vi "SParmSetup_v1.1.vi"(0 "VISA IN":refnum<visa-resource-name>="GPIB0::16::INSTR", 1 "Start Frequency":dbl=10000000.0, 2 "Stop Frequency":dbl=26400000000.0, 3 "Filename":string="MY_MEAS", 5 "Average?":bool=TRUE, 6 "AVG Factor":i32=5, 7 "error in":errorcluster, 8 "Autoscale?":bool, 9 "Trace":i32=1, 10 "Points":dbl=201.0, 11 "Window":i32=1, 12 "IF BW":dbl=1000.0, 13 "Channel":i32=1, 14 "Format":string(combo)="MLINear", 15 "Sweep Type":string(combo)="LINear", 17 "Power Level":dbl=-10.0, 19 "CW Frq.":dbl=1000000000.0, 26 "CW Points":dbl=1.0) -> (20 "VISA Out":refnum<visa-resource-name>="GPIB0::16::INSTR", 27 "error out":errorcluster)   [LabVIEW 2018]
panel:
  in  "Ref Position":i32
  in  "Ref Level":i32
  in  "Scale Per Division":i32=10
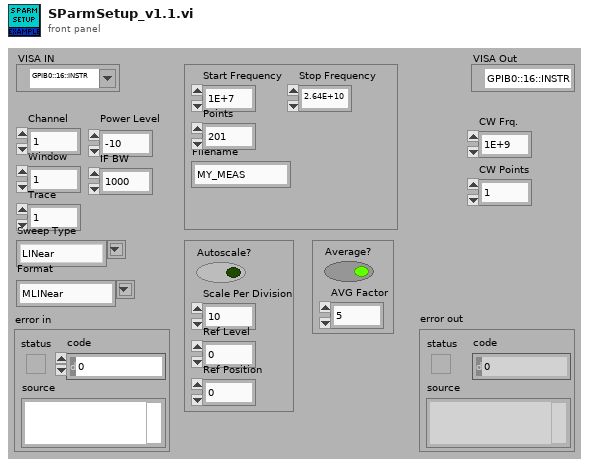
[diagram p1: front panel]
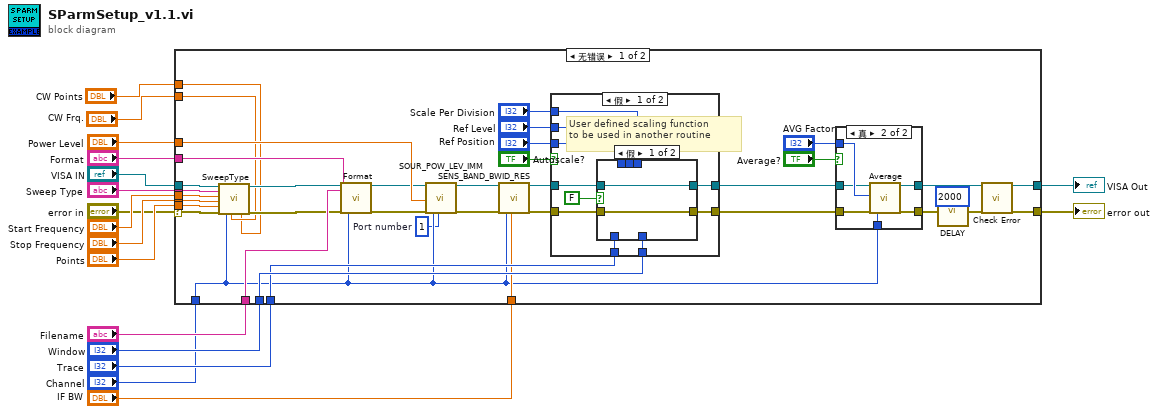
[diagram p0: block diagram]
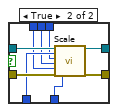
[diagram p3: hidden frame]
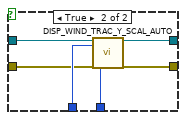
[diagram p4: hidden frame]
diagram:
  n1 = case shown="无错误" "error in" {
    selector: "error in" -> [w23 w92]
    tunnel: [w55 w91] -> w17
    tunnel: [w54 w92] -> w16
    tunnel: "Stop Frequency" -> [w53 _]
    tunnel: "Points" -> [w52 _]
    tunnel: "Sweep Type" -> [w51 _]
    tunnel: "Start Frequency" -> [w50 _]
    tunnel: "Window" -> [w49 _]
    tunnel: "Trace" -> [w48 _]
    tunnel: "VISA IN" -> [w36 w91]
    tunnel: "Power Level" -> [w34 _]
    tunnel: "IF BW" -> [w29 _]
    tunnel: "Filename" -> [w26 _]
    tunnel: "Channel" -> [w25 _]
    tunnel: "Format" -> [w24 _]
    tunnel: "CW Frq." -> [w19 _]
    tunnel: "CW Points" -> [w18 _]
    frame No Error {
      w22 = 1  # Port number
      n2 = call "SweepType.vi"("VISA IN"=w36, "Sweep Type"=w51, "Start Frq."=w50, "Stop Frq."=w53, 4:"Points"=w52, "error in"=w23, "Channel"=w25, "CW Frq."=w19, 13:"Points"=w18) -> ("VISA Out"=w21:refnum<visa-resource-name>, "error out"=w20:errorcluster)  [unwired: 9 in]
      n3 = call "Format.vi"("VISA IN"=w21, "Measurement Name"=w26, "Format"=w24, "error in"=w20, "Channel"=w25) -> ("VISA Out"=w27:refnum<visa-resource-name>, "error out"=w28:errorcluster)  [unwired: 13 in]
      n4 = call "SOUR_POW_LEV_IMM.vi"("VISA IN"=w27, "Power Level"=w34, "error in"=w28, "Channel"=w25, "Port number"=w22) -> ("VISA Out"=w32:refnum<visa-resource-name>, "error out"=w33:errorcluster)  [unwired: 13 in]
      n5 = call "SENS_BAND_BWID_RES.vi"("VISA IN"=w32, "error in"=w33, "Channel"=w25, "Resolution"=w29) -> ("VISA Out"=w31:refnum<visa-resource-name>, "error out"=w30:errorcluster)  [unwired: 14 in]
      n6 = case shown="假" "Autoscale?" {
        tunnel: w30 -> [w72 w87]
        tunnel: w31 -> [w73 w88]
        tunnel: w48 -> [w69 w89]
        tunnel: w49 -> [w68 w90]
        tunnel: [w70 w85] -> w46
        tunnel: [w71 w86] -> w35
        tunnel: "Scale Per Division" -> [w67 _]
        tunnel: "Ref Level" -> [w66 _]
        tunnel: "Ref Position" -> [w65 _]
        frame False {
          # "User defined scaling function\nto be used in another routine"
          n7 = case shown="假" FALSE {
            tunnel: w73 -> [w75 w84]
            tunnel: w72 -> [w74 w83]
            tunnel: [w74 w82] -> w71
            tunnel: [w75 w81] -> w70
            tunnel: w69 -> [_ w80]
            tunnel: w68 -> [_ w79]
            tunnel: w67 -> [_ w78]
            tunnel: w66 -> [_ w77]
            tunnel: w65 -> [_ w76]
            frame False {
            }
            frame True {
              n8 = call "Scale.vi"("VISA IN"=w84, "Trace"=w80, "Scale Per Division"=w78, "Ref Level"=w77, "Ref Position"=w76, "error in"=w83, "Window"=w79) -> ("VISA Out"=w81:refnum<visa-resource-name>, "error out"=w82:errorcluster)  [unwired: 11 in]
            }
          }
        }
        frame True {
          n9 = call "DISP_WIND_TRAC_Y_SCAL_AUTO.vi"("VISA IN"=w88, "Trace"=w89, "error in"=w87, "Window"=w90) -> ("VISA Out"=w85:refnum<visa-resource-name>, "error out"=w86:errorcluster)  [unwired: 14 in]
        }
      }
      n10 = case shown="真" "Average?" {
        tunnel: w46 -> [w57 w58]
        tunnel: w35 -> [w56 w63]
        tunnel: [w56 w62] -> w42
        tunnel: [w57 w61] -> w43
        tunnel: w25 -> [_ w60]
        tunnel: "AVG Factor" -> [_ w59]
        frame False {
        }
        frame True {
          n11 = call "Average.vi"("VISA IN"=w58, "AVG"=w59, "error in"=w63, "Channel"=w60) -> ("VISA Out"=w61:refnum<visa-resource-name>, "error out"=w62:errorcluster)  [unwired: 14 in]
        }
      }
      n12 = call "DELAY.vi"("milliseconds to wait"=u32 2000, "error in (no error)"=w42) -> ("error out"=w41:errorcluster)  [unwired: 13 in]
      n13 = call "Check Error.vi"("VISA Resource Name"=w43, "error in (no error)"=w41) -> ("dup VISA session"=w55:refnum<visa-resource-name>, "error out"=w54:errorcluster)  [unwired: 16 in]
    }
    frame Error {
    }
  }
  "VISA Out" <- w17
  "error out" <- w16
